vi "Constructor.vi"(8 "ErrorIn":errorcluster, 11 "OpenCVFaceDetectionIn":refnum<class "OpenCVFaceDetection.lvclass">) -> (0 "ErrorOut":errorcluster, 3 "OpenCVFaceDetectionOut":refnum<class "OpenCVFaceDetection.lvclass">)   [LabVIEW 2021, in "OpenCVFaceDetection.lvclass"]
doc: "Used to initialize the attributes of the object. This is called at the creation of the object. This VI can be overridden by the child classes to initialize their attributesa"
uses:
  OpenCVFaceDetection.lvclass
  OpenCVFaceDetection.lvclass/OpenCVFaceDetection.ctl
  C:/Localdata/Projects/TriekselSoft/TriekselsoftApplicationFramework/Source/.Externals/Library_EmguCV/Emgu.CV.Platform.NetStandard.dll
  Library_EmguCV/Emgu.CV.Platform.NetStandard.dll
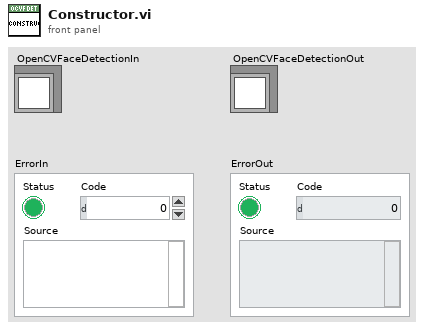
[diagram p1: front panel]
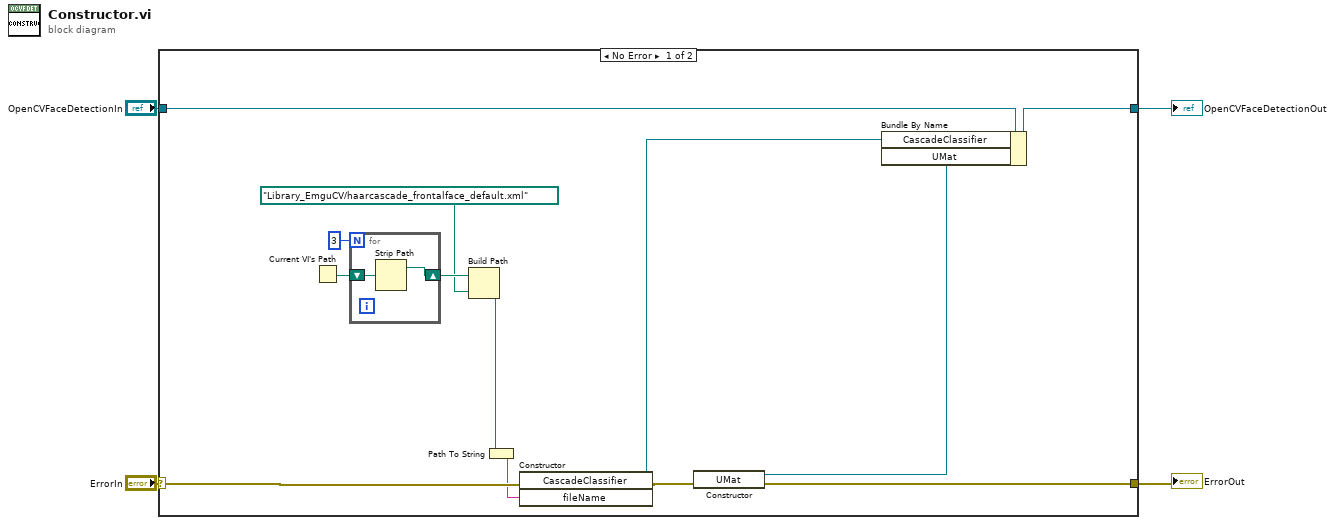
[diagram p0: block diagram]
diagram:
  n1 = case shown="No Error" "ErrorIn" {
    selector: "ErrorIn" -> [w15 w21]
    tunnel: [w17 w21] -> w3
    tunnel: [w14 w20] -> w1
    tunnel: "OpenCVFaceDetectionIn" -> [w11 w20]
    frame No Error {
      n2 = Current VI's Path() -> (path=w10:path)
      n3 = for {
        N: 3 -> [_]
        shift-right: [w18] -> w8
        shift-left: w10 -> [w19]
        n4 = Strip Path(path=w19) -> (stripped path=w18:path)  [unwired: 1 out]
      }
      n5 = Build Path(base path=w8, name or relative path=path "Library_EmguCV/haarcascade_frontalface_default.xml") -> (appended path=w5:path)
      n6 = Path To String(path=w5) -> (string=w6:string)
      n7 = constructor class="CascadeClassifier"(error in=w15, "fileName"=w6) -> (reference out=w12:refnum<k24>, error out=w16:errorcluster)  [unwired: 2 in, 2 out]
      n8 = constructor class="UMat"(error in=w16) -> (reference out=w13:refnum<k24>, error out=w17:errorcluster)  [unwired: 2 in, 1 out]
      n9 = Bundle By Name(cluster=w11, "CascadeClassifier"=w12, "UMat"=w13) -> (w14:refnum<class "OpenCVFaceDetection.lvclass">)
    }
    frame Error {
    }
  }
  "ErrorOut" <- w3
  "OpenCVFaceDetectionOut" <- w1
